vi "ResultSweep.vi"() -> ()   [LabVIEW 2019]
panel:
  out "Module":cluster{dbl[], dbl[]}(graph)
  out "Phase":cluster{dbl[], dbl[]}(graph)
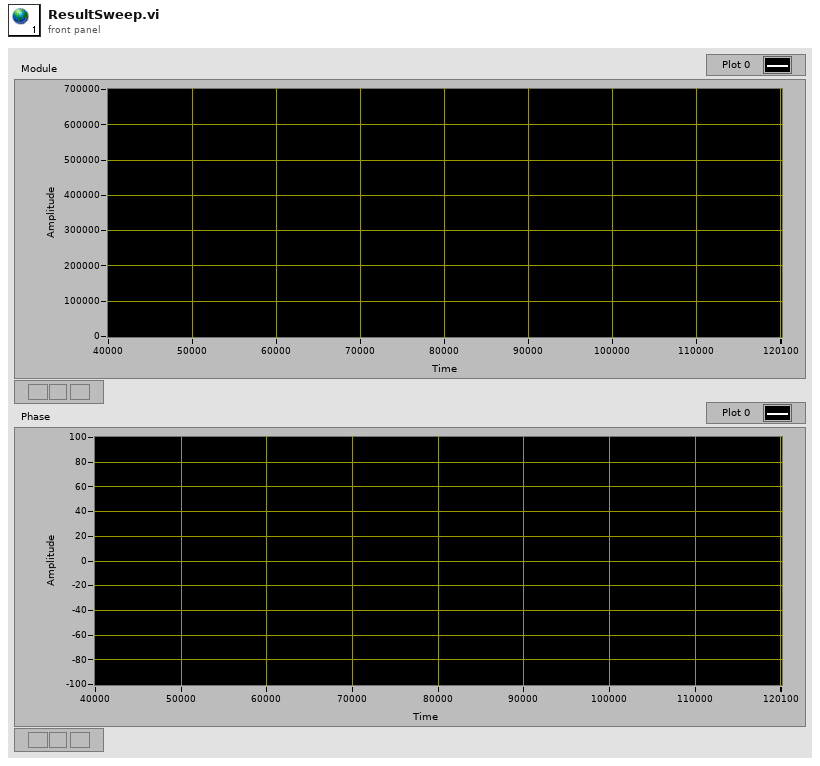
[diagram p1: front panel]
diagram:
